vi "experiment_No.vi"() -> ()   [LabVIEW 2020]
panel:
  in  "experiment_No":i32
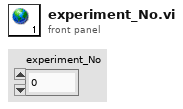
[diagram p1: front panel]
diagram:
